vi "get cluster details.vi"(8 "error in":errorcluster, 10 "Cluster-target":refnum<vi>, 11 "VI Refnum":refnum<vi>) -> (0 "error out":errorcluster, 2 "Control details":string)   [LabVIEW 2020, in "ui-testing.lvlib"]
uses:
  ui-testing.lvlib
  <vilib>/Utility/traverseref.llb/TRef TravTarget.ctl
  <vilib>/Utility/traverseref.llb/VI Scripting - Traverse.lvlib
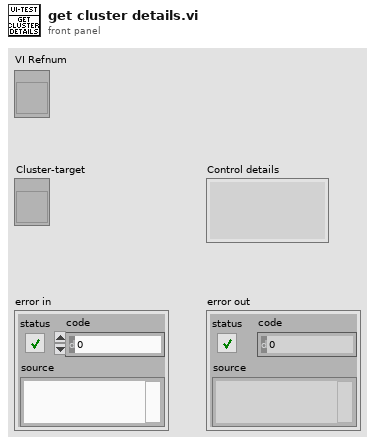
[diagram p1: front panel]
types:
  T1 = typedef "TRef TravTarget.ctl" = enum16{"FP", "BD", "Other"}
  T2 = cluster{"Caption":string, "Label":string, "Visible":bool}
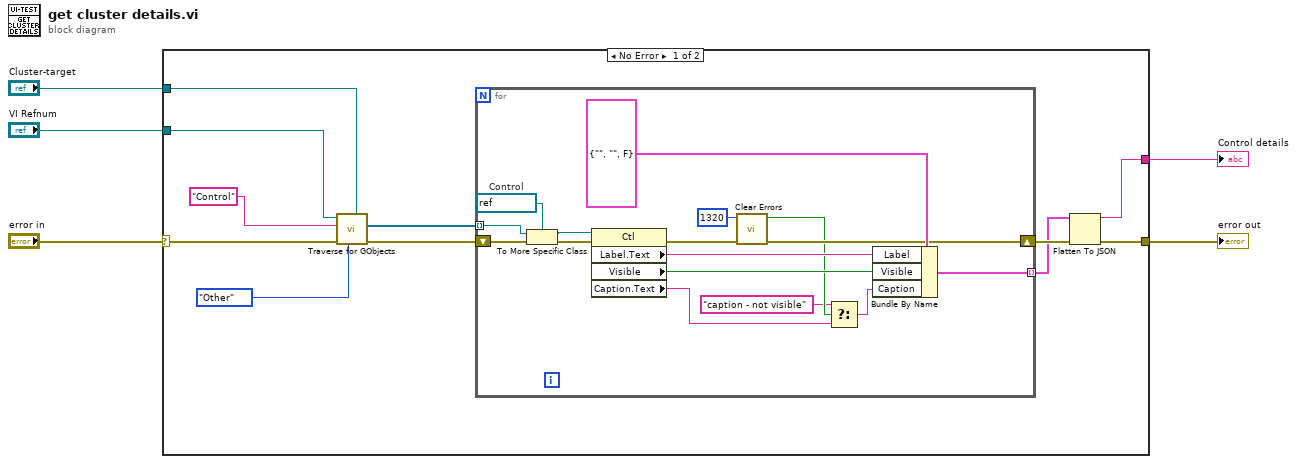
[diagram p0: block diagram]
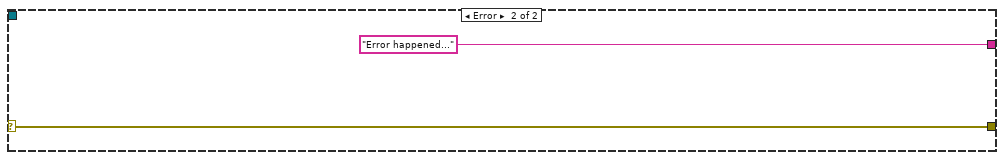
[diagram p2: hidden frame]
diagram:
  n1 = case shown="No Error" "error in" {
    selector: "error in" -> [w9 w34]
    tunnel: [w15 w34] -> w1
    tunnel: [w13 "Error happened..."] -> w5
    tunnel: "VI Refnum" -> [w7 _]
    tunnel: "Cluster-target" -> [w6 _]
    frame No Error {
      n2 = call <vilib>:"Traverse for GObjects.vi"("Other Refnum"=w6, "Traverse Target"=TRef_TravTarget."Other", "error in (no error)"=w9, "Class Name"="Control", "VI Refnum"=w7) -> ("error out"=w8:errorcluster, "References"=w10:refnum<vi>[])  [unwired: 3 in, 2 out]
      n3 = for {
        tunnel: [w28] -> w14 mode=indexing
        shift-right: [w26] -> w16
        shift-left: w8 -> [w32]
        tunnel: w10 -> [w19] mode=indexing
        w17 = refnum<vi> refnum  # Control
        n4 = To More Specific Class(target class=w17, reference=w19, error in=w32) -> (specific class reference=w18:refnum<vi>, error out=w20:errorcluster)
        n5 = property class="Ctl"(reference=w18, error in=w20) -> (error out=w27:errorcluster, "Label.Text"=w31:string, "Visible"=w30:bool, "Caption.Text"=w24:string)  [unwired: 1 out]
        n6 = call <vilib>:"Clear Errors.vi"("error in (no error)"=w27, "specific error code to clear (0: all)"=1320) -> ("error out"=w26:errorcluster, "specific error cleared?"=w22:bool)  [unwired: 4 in]
        n7 = Select(t="caption - not visible", s=w22, f=w24) -> (s? t:f=w23:string)
        n8 = Bundle By Name(cluster=T2 {"Caption"="", "Label"="", "Visible"=FALSE}, "Label"=w31, "Visible"=w30, "Caption"=w23) -> (w28:T2)
      }
      n9 = Flatten To JSON(anything=w14, error in (no error)=w16) -> (JSON string=w13:string, 11:w15:errorcluster)  [unwired: 1 in]
    }
    frame Error {
    }
  }
  "Control details" <- w5
  "error out" <- w1
